vi "Database-ExportData.vi"(7 "Idx":i32, 8 "error in":errorcluster, 10 "Result in":T1) -> (0 "error out":errorcluster, 2 "Result out":T1, 4 "Export time":timestamp)   [LabVIEW 2016]
doc: "Go to DB->WriteStationValues action\nReturn boolean flag to show if data was saved to DB successfully\n\nWabco 2017 All right reserved\nAuthor: maciej.szupienko@wabco-auto.com"
uses:
  Cache/Cache.TestSteps.Fglb.ResultData.ctl
  ProdaNG/Controls/ProdaNG.ProcessResult.ctl
  ProdaNG/Controls/ProdaNG.ProcessStepResult.ctl
  ProdaNG/Controls/ProdaNG.TestStepResult.ctl
  ProdaNG/Controls/ProdaNG.TestValueResult.ctl
  Database.Action.ctl
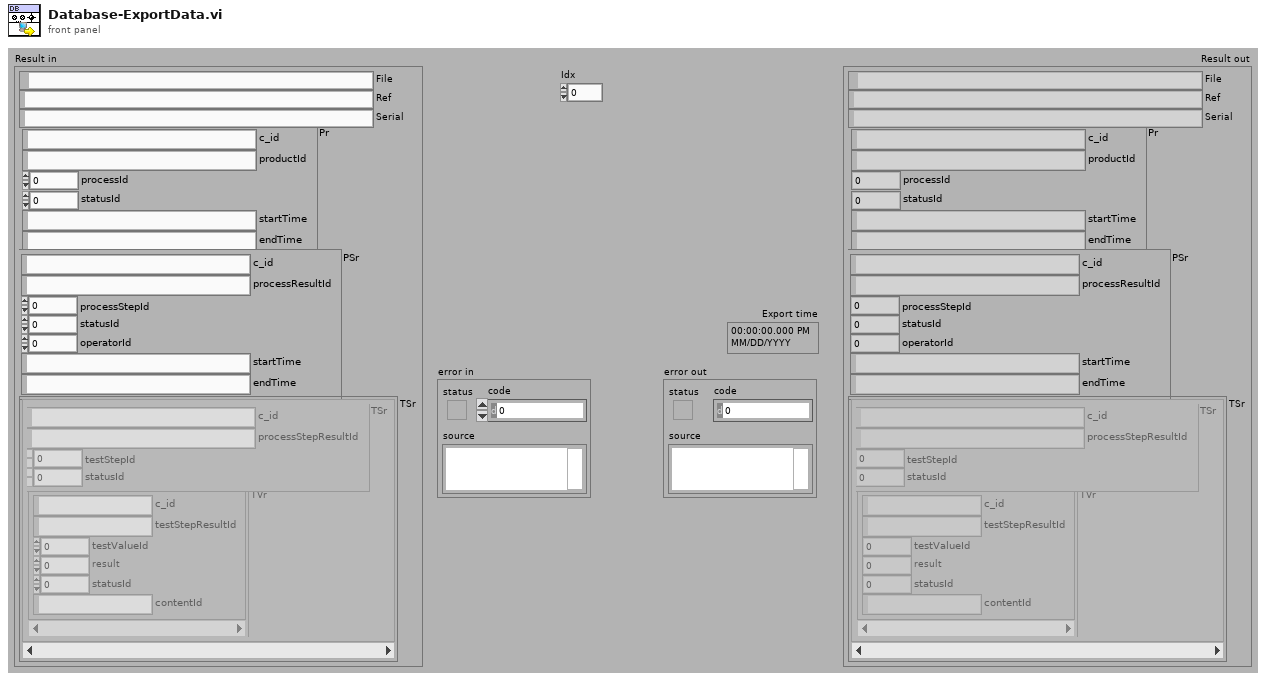
[diagram p1: front panel]
types:
  T1 = typedef "Cache.TestSteps.Fglb.ResultData.ctl" = cluster{"File":path, "Ref":string, "Serial":string, "Pr":T2, "PSr":T3, "TSr":cluster{"TSr":T4, "TVr":T5[]}[]}
  T2 = typedef "ProdaNG.ProcessResult.ctl" = cluster{"c_id":string, "productId":string, "processId":i32, "statusId":i32, "startTime":string, "endTime":string}
  T3 = typedef "ProdaNG.ProcessStepResult.ctl" = cluster{"c_id":string, "processResultId":string, "processStepId":i32, "statusId":i32, "operatorId":i32, "startTime":string, "endTime":string}
  T4 = typedef "ProdaNG.TestStepResult.ctl" = cluster{"c_id":string, "processStepResultId":string, "testStepId":i32, "statusId":i32}
  T5 = typedef "ProdaNG.TestValueResult.ctl" = cluster{"c_id":string, "testStepResultId":string, "testValueId":i32, "result":dbl, "statusId":i32, "contentId":string}
  T6 = typedef "Database.Action.ctl" = enum32{"idle", "constructor", "destructor", "--- DB ---", "Setup", "Disconnect", "Connect", "GetAllStatuses"}
  T7 = cluster{"Result in":T1, "Export time":timestamp, "error IO":errorcluster}
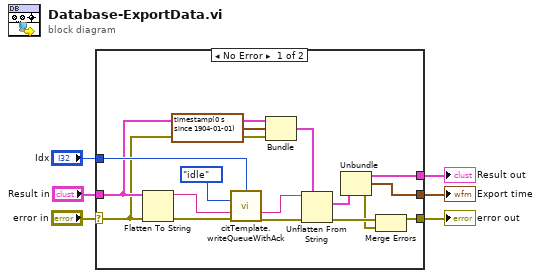
[diagram p0: block diagram]
diagram:
  n1 = case shown="No Error" "error in" {
    selector: "error in" -> [w10 w23]
    tunnel: [w7 w23] -> w5
    tunnel: "Idx" -> [w21 _]
    tunnel: "Result in" -> [w15 _]
    tunnel: [w11 _] -> w2
    tunnel: [w9 _] -> w1
    frame No Error {
      n2 = Flatten To String(anything=w15, error in (no error)=w10) -> (data string=w17:string, error out=w18:errorcluster)  [unwired: 2 in, 1 out]
      n3 = call "citTemplate.writeQueueWithAck.vi"("instance (0)"=w21, "event in"=Database.Action."idle" ("Action"), "(flatten) data in"=w17, "error in (no error)"=w18) -> ("notification data"=w16:string, "error out"=w20:errorcluster)  [unwired: 9 in, 1 out]
      n4 = Bundle("Result in"=w15, "Export time"=timestamp(0 s since 1904-01-01), "error IO"=w10) -> (w13:T7)  [unwired: 1 in]
      n5 = Unflatten From String(type=w13, binary string=w16, error in (no error)=w20) -> (value=w12:T7, error out=w19:errorcluster)  [unwired: 2 in, 1 out]
      n6 = Unbundle(w12) -> ("Result in"=w11:T1, "Export time"=w9:timestamp, "error IO"=w8:errorcluster)
      n7 = Merge Errors(w19, w8) -> (w7:errorcluster)
    }
    frame Error {
    }
  }
  "error out" <- w5
  "Result out" <- w2
  "Export time" <- w1
